vi "Read Project.vi"(8 "error in (no error)":errorcluster, 11 "Editor in":refnum<class "Editor.lvclass">) -> (0 "error out":errorcluster, 2 "Project.lvclass":refnum<class "Project.lvclass">, 3 "Editor out":refnum<class "Editor.lvclass">)   [LabVIEW 2015, in "Editor.lvclass"]
uses:
  Editor.lvclass
  Project.lvclass
  Editor.lvclass/Editor.ctl
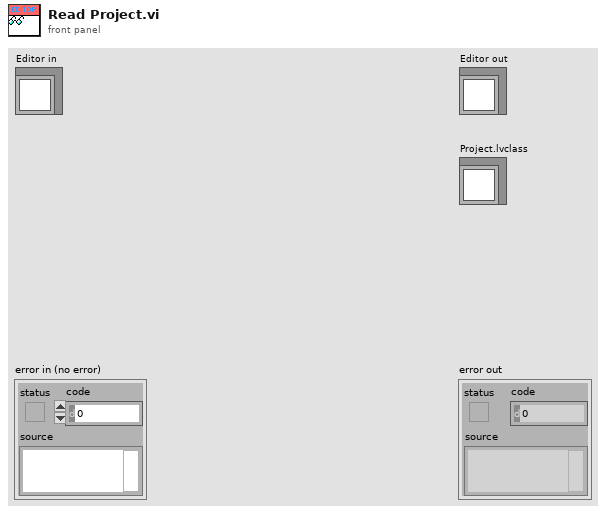
[diagram p1: front panel]
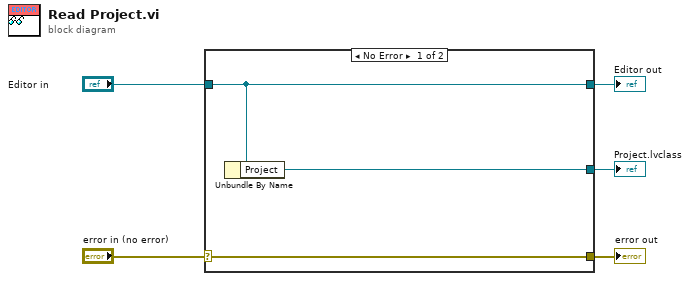
[diagram p0: block diagram]
diagram:
  n1 = case shown="No Error" "error in (no error)" {
    selector: "error in (no error)" -> [w8 w9]
    tunnel: [w8 w9] -> w4
    tunnel: [w7 w10] -> w2
    tunnel: "Editor in" -> [w7 w10]
    tunnel: [w6 _] -> w1
    frame No Error {
      n2 = Unbundle By Name(w7) -> ("Project"=w6:refnum<class "Project.lvclass">)
    }
    frame Error {
    }
  }
  "error out" <- w4
  "Editor out" <- w2
  "Project.lvclass" <- w1
